vi "Config - Search.vi"(8 "error in (no error)":errorcluster, 10 "Account Number":u32, 11 "Config Array":T2 {"Balance" format="%9.2g"}) -> (0 "error out":errorcluster, 2 "Account Exist?":bool, 3 "Config Data":T1 {"Balance" format="%9.2g"})   [LabVIEW 2017]
doc: "Provides SEARCH mechanism in Config Array by Account Number."
uses:
  Controls/Config Array.ctl
  Controls/Config Data.ctl
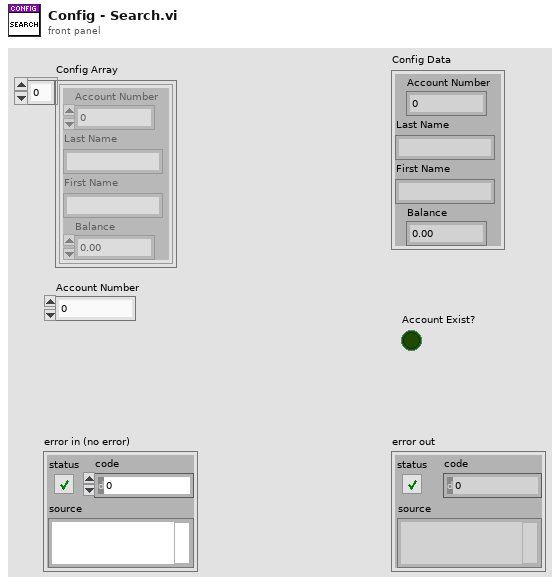
[diagram p1: front panel]
types:
  T1 = typedef "Config Data.ctl" = cluster{"Account Number":u32, "Last Name":string, "First Name":string, "Balance":dbl}
  T2 = typedef "Config Array.ctl" = T1[]
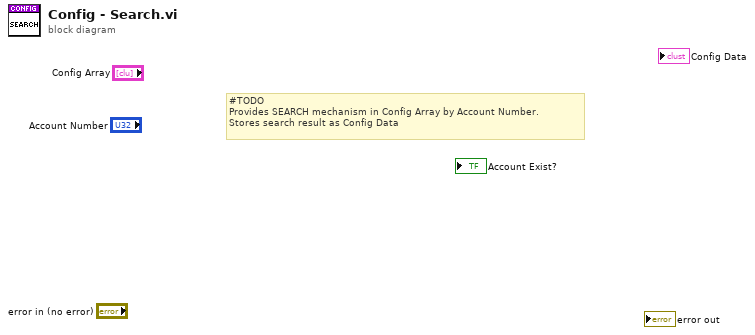
[diagram p0: block diagram]
diagram:
  # "#TODO\nProvides SEARCH mechanism in Config Array by Account Number.\nStores search result as Config Data"
